vi "Diagnostic Logger v1.5.vi"   [LabVIEW 2014]
uses:
  <vilib>/Rock Robotics/WPI/DriverStation/WPI_DriverStationRobotMode2.ctl
  <vilib>/Utility/file.llb/Write To Spreadsheet File (DBL).vi
  Begin/Global Variables.vi
panel:
  # "CSV Columns Transposed:\n\nRobot Mode (0=?, 1=Auton, 2=Teleop)\nElapsed Time (ms)\ndt (ms)\nGyro Yaw\nGyro Pitch\nGyro Roll\nDriver JS LX\nDriver JS LY\nDriver JS RX\nDrive Resolver FL\nDrive Resolver FR\nDrive Resolver BL\nDrive Resolver BR\nDrive Encoder FL\nDrive Encoder FR\nDrive Encoder BL\nDrive Encoder BR\nDrive Speed FL\nDrive Speed FR\nDrive Speed BL\nDrive Speed BR\nLift Height Left\nLift Height Right\nLift Rate Left\nLift Rate Right"
  # "Data Usage Rates:\n\n20 KB / sec\n1.2 MB / min\n72 MB / hour"
types:
  T1 = typedef "WPI_DriverStationRobotMode2.ctl" = enum16{"Autonomous Disabled", "Autonomous Enabled", "Teleop Disabled", "Teleop Enabled", "Disconnected", "Finish", "Test Disabled", "Test Enabled", "Emergency Stopped"}
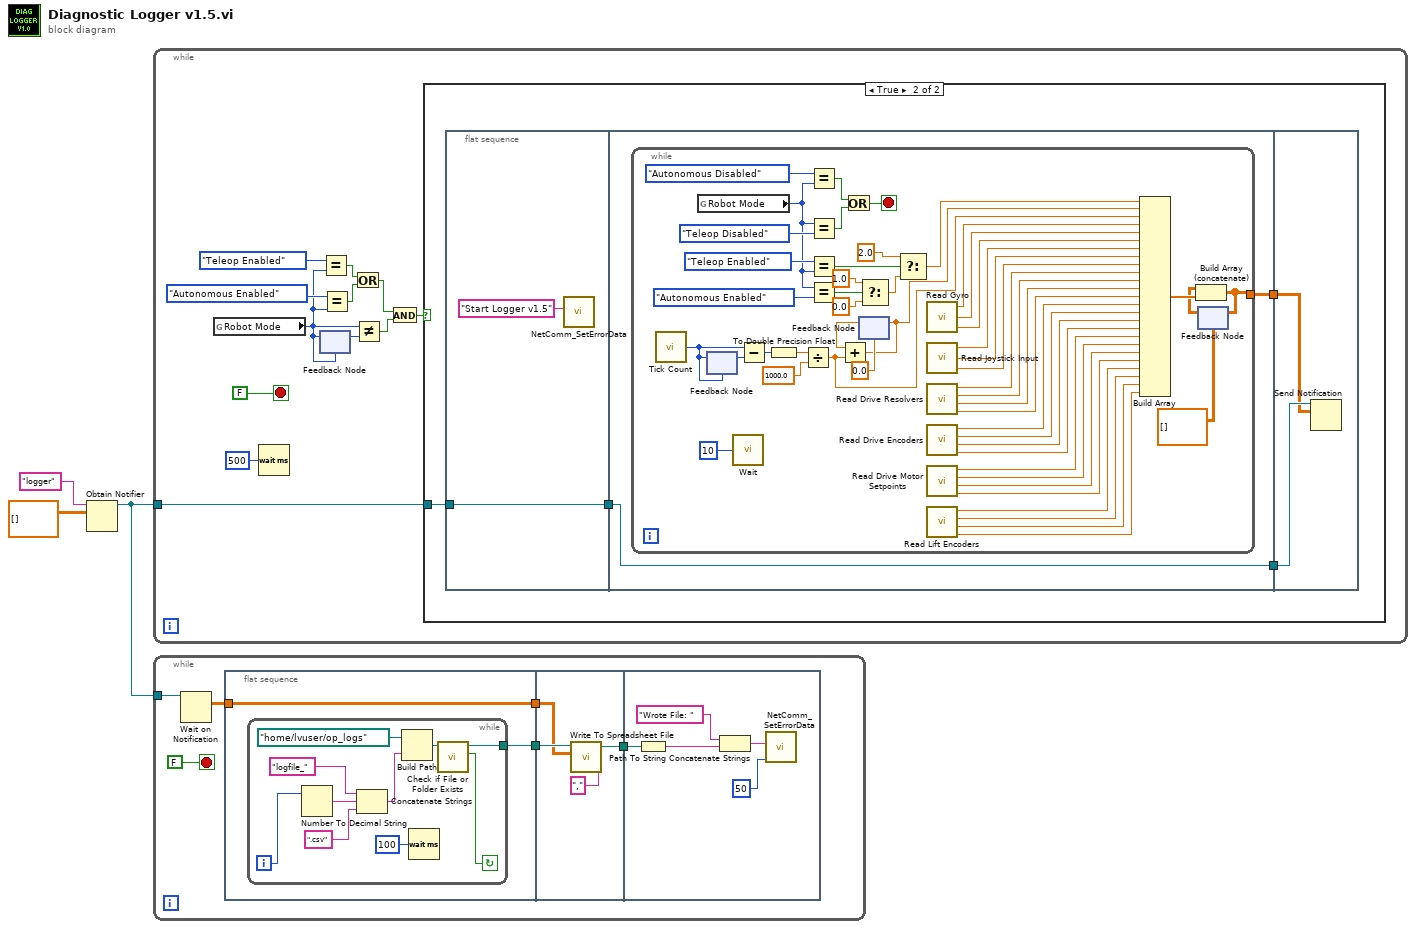
[diagram p0: block diagram]
diagram:
  n1 = Obtain Notifier(name (unnamed)="logger", notification data type=dbl[][] []) -> (notifier out=w1:refnum<notifier>)  [unwired: 2 in, 2 out]
  n2 = while {
    tunnel: w1 -> [w4]
    stop <- FALSE stop-if-true
    n3 = global read "Global Variables.vi" "Robot Mode"() -> (w10:T1)
    n4 = Wait (ms)(milliseconds to wait=u32 500) -> ()  [unwired: 1 out]
    n5 = feedback-in #1(w10) -> ()
    n6 = feedback #1(w10) -> (w14:T1)
    n7 = Equal?(x=WPI_DriverStationRobotMode2."Teleop Enabled", y=w10) -> (x = y?=w9:bool)
    n8 = Equal?(x=WPI_DriverStationRobotMode2."Autonomous Enabled", y=w10) -> (x = y?=w8:bool)
    n9 = Or(x=w9, y=w8) -> (x .or. y?=w7:bool)
    n10 = Not Equal?(x=w10, y=w14) -> (x != y?=w13:bool)
    n11 = And(x=w7, y=w13) -> (x .and. y?=w6:bool)
    n12 = case shown="True" w6 {
      tunnel: w4 -> [_ w19]
      frame False {
      }
      frame True {
        n13 = flat-sequence {
          tunnel: w19 -> [w20]
          tunnel: [w20] -> w18
          tunnel: w18 -> [w23]
          tunnel: [w23] -> w17
          tunnel: [w22] -> w16
          tunnel: w17 -> [w76]
          tunnel: w16 -> [w75]
          frame #0 {
            n14 = call <vilib>:"NetComm_SetErrorData.vi"("Error Data"="Start Logger v1.5") -> ()  [unwired: 3 in, 8 out]
          }
          frame #1 {
            n15 = while {
              tunnel: [w24] -> w22
              stop <- w56 stop-if-true
              n16 = call "Tick Count"() -> ("Tick Count(uSec)"=w74:u32)
              n17 = global read "Global Variables.vi" "Robot Mode"() -> (w62:T1)
              n18 = feedback-in #2(w74) -> ()
              n19 = feedback #2(w74) -> (w73:u32)
              n20 = call "Wait"("Count(mSec)"=u32 10) -> ()  [unwired: 1 out]
              n21 = Subtract(x=w74, y=w73) -> (x-y=w55:u32)
              n22 = To Double Precision Float(number=w55) -> (double precision float=w54:dbl)
              n23 = Divide(x=w54, y=1000.0) -> (x/y=w50:dbl)
              n24 = Equal?(x=WPI_DriverStationRobotMode2."Autonomous Disabled", y=w62) -> (x = y?=w66:bool)
              n25 = Equal?(x=w62, y=WPI_DriverStationRobotMode2."Teleop Disabled" ("x")) -> (x = y?=w67:bool)
              n26 = Equal?(x=WPI_DriverStationRobotMode2."Teleop Enabled", y=w62) -> (x = y?=w64:bool)
              n27 = Equal?(x=w62, y=WPI_DriverStationRobotMode2."Autonomous Enabled" ("x")) -> (x = y?=w61:bool)
              n28 = Or(x=w66, y=w67) -> (x .or. y?=w56:bool)
              n29 = feedback #3(0.0) -> (w70:dbl)
              n30 = Add(x=w70, y=w50) -> (x+y=w51:dbl)
              n31 = feedback-in #3(w51) -> ()
              n32 = Select(t=1.0, s=w61, f=0.0) -> (s? t:f=w60:dbl)
              n33 = Select(t=2.0, s=w64, f=w60) -> (s? t:f=w52:dbl)
              n34 = call "Read Gyro.vi"() -> ("Roll"=w47:dbl, "Pitch"=w48:dbl, "Yaw"=w49:dbl)
              n35 = call "Read Joystick Input.vi"() -> ("Driver Joystick X2"=w44:dbl, "Driver Joystick Y1"=w45:dbl, "Driver Joystick X1"=w46:dbl)
              n36 = call "Read Drive Resolvers.vi"() -> ("Drive Resolver BR"=w40:dbl, "Drive Resolver BL"=w41:dbl, "Drive Resolver FR"=w42:dbl, "Drive Resolver FL"=w43:dbl)
              n37 = call "Read Drive Encoders.vi"() -> ("Drive Encoder BR"=w36:dbl, "Drive Encoder BL"=w37:dbl, "Drive Encoder FR"=w38:dbl, "Drive Encoder FL"=w39:dbl)
              n38 = call "Read Drive Motor Setpoints.vi"() -> ("Drive BR Setspeed"=w32:dbl, "Drive BL Setspeed"=w33:dbl, "Drive FR Setspeed"=w34:dbl, "Drive FL Setspeed"=w35:dbl)
              n39 = call "Read Lift Encoders.vi"() -> ("Lift Right Rate [counts/sec]"=w28:dbl, "Lift Left Rate [counts/sec]"=w29:dbl, "Lift Right Height [counts]"=w30:dbl, "Lift Left Height [counts]"=w31:dbl)
              n40 = Build Array(w52, w51, w50, w49, w48, w47, w46, w45, w44, w43, w42, w41, w40, w39, w38, w37, w36, w35, w34, w33, w32, w31, w30, w29, w28) -> (w27:dbl[])
              n41 = feedback #4(dbl[][] []) -> (w26:dbl[][])
              n42 = Build Array (concatenate)(w26, w27) -> (w24:dbl[][])
              n43 = feedback-in #4(w24) -> ()
            }
          }
          frame #2 {
            n44 = Send Notification(notification=w75, notifier=w76) -> ()  [unwired: 1 in, 2 out]
          }
        }
      }
    }
  }
  n45 = while {
    tunnel: w1 -> [w82]
    stop <- FALSE stop-if-true
    n46 = Wait on Notification(notifier=w82) -> (notification=w80:dbl[][])  [unwired: 3 in, 3 out]
    n47 = flat-sequence {
      tunnel: w80 -> [w84]
      tunnel: [w84] -> w79
      tunnel: [w83] -> w78
      tunnel: w79 -> [w96]
      tunnel: w78 -> [w97]
      tunnel: [w95] -> w77
      tunnel: w77 -> [w99]
      frame #0 {
        n48 = while {
          tunnel: [w87] -> w83
          i -> [w86]
          stop <- w94 continue-if-true
          n49 = Number To Decimal String(number=w86) -> (decimal integer string=w91:string)  [unwired: 1 in]
          n50 = Concatenate Strings("logfile_", w91, ".csv") -> (w90:string)
          n51 = Build Path(base path=path "/home/lvuser/op_logs" ("file path (dialog if empty)"), name or relative path=w90) -> (appended path=w93:path)
          n52 = Wait (ms)(milliseconds to wait=u32 100) -> ()  [unwired: 1 out]
          n53 = call <vilib>:"Check if File or Folder Exists.vi"("path"=w93) -> ("file or folder exists?"=w94:bool, "dup path"=w87:path)  [unwired: 8 in, 1 out]
        }
      }
      frame #1 {
        n54 = call-poly <vilib>:"Write To Spreadsheet File.vi"("delimiter (\\t)"="," ("delimiter (\\t)"), "2D data"=w96, "file path (dialog if empty)"=w97) -> ("new file path (Not A Path if cancelled)"=w95:path)  [unwired: 5 in]
      }
      frame #2 {
        n55 = Path To String(path=w99) -> (string=w100:string)
        n56 = Concatenate Strings("Wrote File: ", w100) -> (w102:string)
        n57 = call <vilib>:"NetComm_SetErrorData.vi"("Timeout (ms)"=50, "Error Data"=w102) -> ()  [unwired: 2 in, 8 out]
      }
    }
  }
